vi "Create Icon Layer.vi"(8 "error in (no error)":errorcluster, 9 "Template data":T5 {"Opacity" scale=0.0..100.0}, 10 "Icon data":T1={"Text Visible?"=FALSE, "Text Opacity"=0, "Templ Visible?"=FALSE, "Templ Opacity"=0, "Relative Path from 1 to 2"=path "", "Image"=bytes[0], "All User Layers"=[], "Body Text"={"Line 1 text"="", "Line 2 text"="", "Line 3 text"="", "Line 4 text"="", "Line 1 color"=0, "Line 2 color"=0, "Line 3 color"=0, "Line 4 color"=0, "Body Text Spec"={"Font"="", "Alignment"=0, "Size"=3}, "Center text vertically"=FALSE, "Capitalize Text"=FALSE}} {"Body Text"."Body Text Spec"."Alignment" items=["left", "center", "right"]}, 11 "Text data":T5 {"Opacity" scale=0.0..100.0}) -> (0 "error out":errorcluster, 3 "Icon out":refnum<class "Icon.lvclass">)   [LabVIEW 2017, in "LabVIEW Icon API.lvlib"]
doc: "Create an Icon Layer with the given data from the LabVIEW Icon Data."
uses:
  <vilib>/LabVIEW Icon API/LabVIEW Icon API.lvlib
  <vilib>/LabVIEW Icon API/lv_icon/Controls/Layer.ctl
  <vilib>/LabVIEW Icon API/lv_icon/Classes/Icon/Icon.lvclass
  <vilib>/LabVIEW Icon API/lv_icon/Controls/LabVIEW Icon Stored Information.ctl
  <vilib>/LabVIEW Icon API/lv_icon/Classes/Layer/Layer.lvclass
  <vilib>/LabVIEW Icon API/lv_icon/Controls/BodyText.ctl
  <vilib>/LabVIEW Icon API/lv_icon/Controls/Font.ctl
  <vilib>/LabVIEW Icon API/lv_icon/Controls/Alignment.ctl
  <vilib>/LabVIEW Icon API/lv_icon/Controls/LayerType.ctl
  <vilib>/LabVIEW Icon API/lv_icon/Classes/Icon Framework/Icon Framework.lvclass
  <vilib>/LabVIEW Icon API/lv_icon/Controls/Graphic.ctl
  <vilib>/LabVIEW Icon API/lv_icon/lv_icon.lvlib
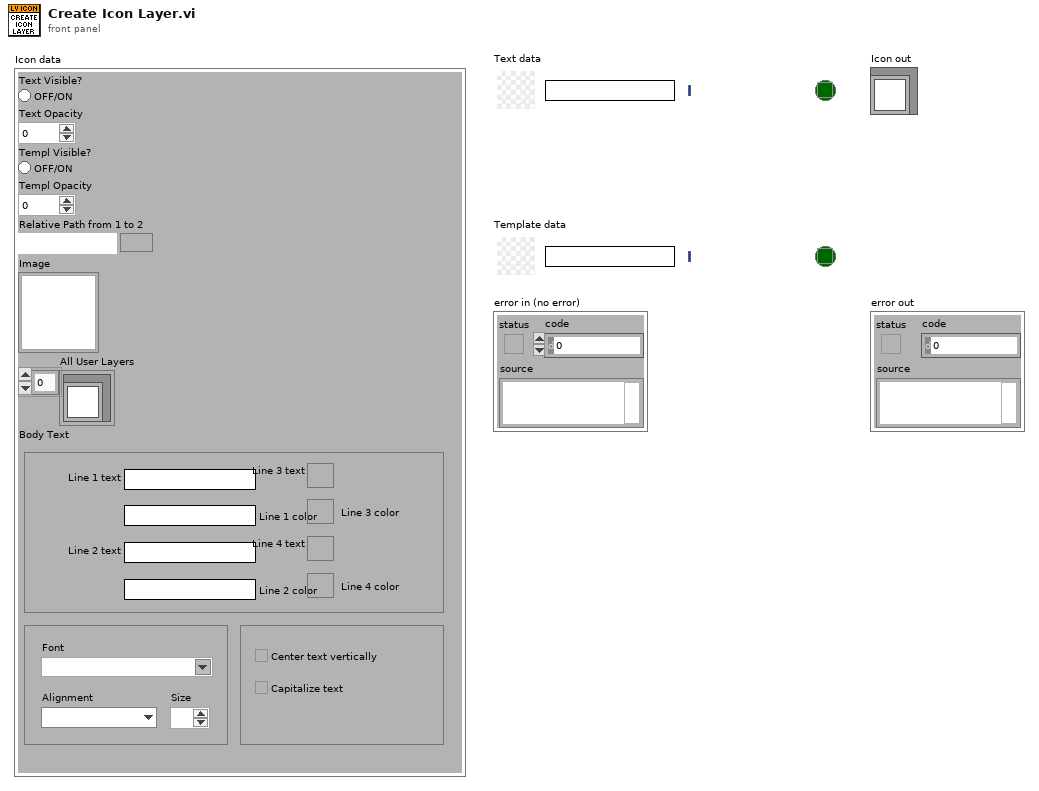
[diagram p1: front panel]
types:
  T1 = typedef "LabVIEW Icon Stored Information.ctl" = cluster{"Text Visible?":bool, "Text Opacity":u8, "Templ Visible?":bool, "Templ Opacity":u8, "Relative Path from 1 to 2":path, "Image":picture, "All User Layers":refnum<class "Layer.lvclass">[], "Body Text":T2}
  T2 = typedef "BodyText.ctl" = cluster{"Line 1 text":string, "Line 2 text":string, "Line 3 text":string, "Line 4 text":string, "Line 1 color":u32, "Line 2 color":u32, "Line 3 color":u32, "Line 4 color":u32, "Body Text Spec":cluster{"Font":T3, "Alignment":T4, "Size":u8}, "Center text vertically":bool, "Capitalize Text":bool}
  T3 = typedef "Font.ctl" = string
  T4 = typedef "Alignment.ctl" = u16
  T5 = typedef "Layer.ctl" = cluster{"LayerIcon":picture, "LayerName":string, "Opacity":u8, "Visibility?":bool}
  T6 = typedef "Graphic.ctl" = cluster{"Rectangle":cluster{"left":i16, "top":i16, "right":i16, "bottom":i16}, "Path":path, "Image":picture, "Filter":string, "FileName":string}
  T7 = typedef "LayerType.ctl" = enum16{"Graphic", "Text", "Tool", "Graphic Drop"}
  T8 = typedef "imagedata.ctl" = cluster{"image type":i32, "image depth":i32, "image":u8[], "mask":u8[], "colors":u32[], "Rectangle":cluster{"left":i16, "top":i16, "right":i16, "bottom":i16}}
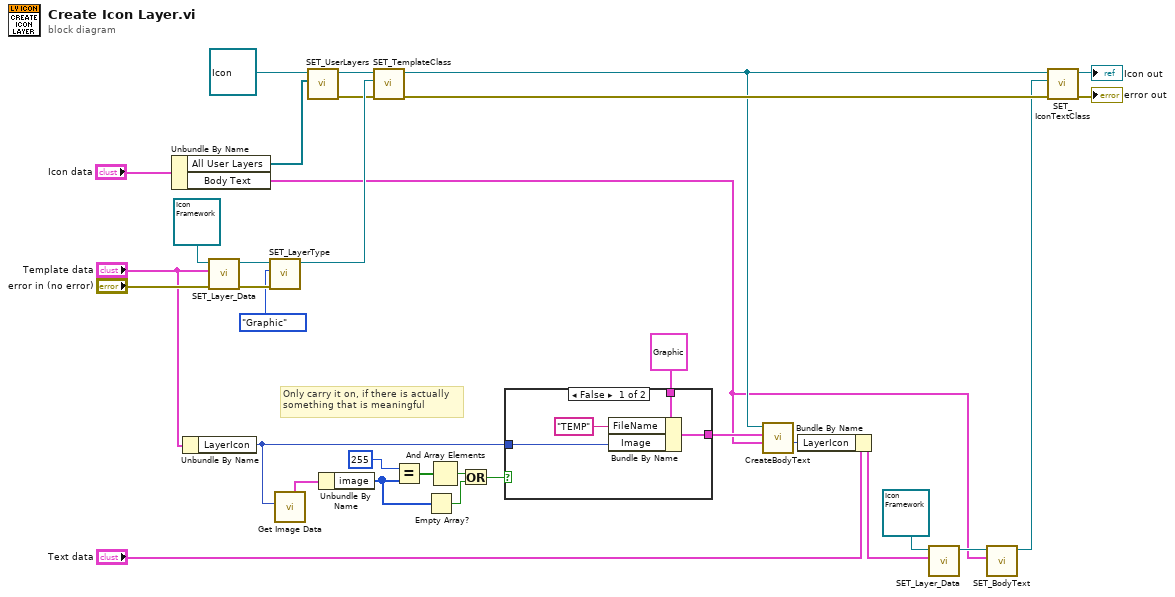
[diagram p0: block diagram]
diagram:
  # "Only carry it on, if there is actually\nsomething that is meaningful"
  n1 = Unbundle By Name("Icon data") -> ("All User Layers"=w23:refnum<class "Layer.lvclass">[], "Body Text"=w13:T2)
  n2 = Unbundle By Name("Template data") -> ("LayerIcon"=w3:picture)
  n3 = call-dynamic "SET_Layer_Data.vi"("error in (no error)"="error in (no error)", "Data"="Template data", "Layer.lvclass in"=refnum<class "Icon Framework.lvclass"> refnum ("lv_icon.lvlib:Icon Framework.lvclass")) -> ("error out"=w32:errorcluster, "Layer.lvclass out"=w29:refnum<class "Icon Framework.lvclass">)  [unwired: 1 in, 6 out]
  n4 = call-dynamic "SET_LayerType.vi"("error in (no error)"=w32, "Type"=LayerType."Graphic", "Layer.lvclass in"=w29) -> ("Layer.lvclass out"=w28:refnum<class "Icon Framework.lvclass">)  [unwired: 8 out]
  n5 = call <vilib>:"Get Image Data.vi"("Pic In"=w3) -> ("image data out"=w9:T8)  [unwired: 2 in, 8 out]
  n6 = call-dynamic "SET_UserLayers.vi"("Layers"=w23, "Icon.lvclass in"=refnum<class "Icon.lvclass"> refnum ("Icon in")) -> ("error out"=w26:errorcluster, "Icon.lvclass out"=w27:refnum<class "Icon.lvclass">)  [unwired: 8 in]
  n7 = Unbundle By Name(w9) -> ("image"=w5:u8[])
  n8 = call-dynamic "SET_TemplateClass.vi"("error in (no error)"=w26, "Icon Framework.lvclass"=w28, "Icon.lvclass in"=w27) -> ("error out"=w20:errorcluster, "Icon.lvclass out"=w19:refnum<class "Icon.lvclass">)  [unwired: 7 out]
  n9 = Equal?(x=u8 255, y=w5) -> (x = y?=w7:bool[])
  n10 = Empty Array?(array=w5) -> (empty?=w4:bool)
  n11 = And Array Elements(Boolean array=w7) -> (logical AND=w6:bool)
  n12 = Or(x=w6, y=w4) -> (x .or. y?=w2:bool)
  n13 = case shown="False" w2 {
    tunnel: [w37 w38] -> w17
    tunnel: w3 -> [w36 _]
    tunnel: T6 {"Rectangle"={"left"=0, "top"=0, "right"=0, "bottom"=0}, "Path"=path "", "Image"=bytes[0], "Filter"="", "FileName"=""} ("Path and Icon Template") -> [w35 w38]
    frame False {
      n14 = Bundle By Name(cluster=w35, "FileName"="TEMP", "Image"=w36) -> (w37:T6)
    }
    frame True {
    }
  }
  n15 = call <vilib>:"CreateBodyText.vi"("Body Text"=w13, "Path and Icon Template"=w17, "Icon.lvclass in"=w19) -> ("Body Text"=w14:picture)  [unwired: 8 in]
  n16 = Bundle By Name(cluster="Text data", "LayerIcon"=w14) -> (w15:T5)
  n17 = call-dynamic "SET_Layer_Data.vi"("Data"=w15, "Layer.lvclass in"=refnum<class "Icon Framework.lvclass"> refnum ("lv_icon.lvlib:Icon Framework.lvclass")) -> ("Layer.lvclass out"=w22:refnum<class "Icon Framework.lvclass">)  [unwired: 8 in, 1 out]
  n18 = call-dynamic "SET_BodyText.vi"("Body Text"=w13, "Icon Framework.lvclass in"=w22) -> ("Icon Framework.lvclass out"=w12:refnum<class "Icon Framework.lvclass">)  [unwired: 8 in, 1 out]
  n19 = call-dynamic "SET_IconTextClass.vi"("error in (no error)"=w20, "Icon Framework.lvclass"=w12, "Icon.lvclass in"=w19) -> ("error out"=→"error out":errorcluster, "Icon.lvclass out"=→"Icon out":refnum<class "Icon.lvclass">)  [unwired: 7 out]
